vi "write digital out.vi"(8 "error in (no error)":errorcluster) -> ()   [LabVIEW 2015]
uses:
  <vilib>/Rock Robotics/SystemInterfaces/DIO/FPGA_DIOChannel.ctl
  <vilib>/Platform/TimedLoop/XDataNode/timing_clust.ctl
  <vilib>/Platform/TimedLoop/XDataNode/nitl_modes.ctl
  <vilib>/Platform/TimedLoop/XDataNode/wakeup.ctl
  <vilib>/Rock Robotics/WPI/Counter/WPI_CounterDigitalInputToDigitalSource.vi
  <vilib>/Rock Robotics/WPI/Counter/WPI_CounterOpen UpDown Mode.vi
  <vilib>/platform/TimedLoop/XDataNode/XDataNode.xnode
  <vilib>/Platform/TimedLoop/XDataNode/XDNodeRunTimeDep.lvlib
panel:
  out "Value 2":i32
  out "Value":bool
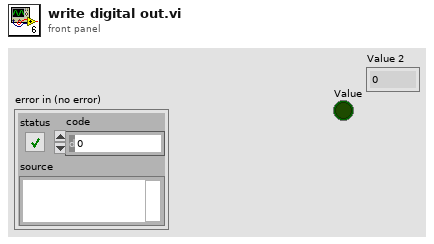
[diagram p1: front panel]
types:
  T1 = typedef "FPGA_DIOChannel.ctl" = enum8{"DIO 0", "DIO 1", "DIO 2", "DIO 3", "DIO 4", "DIO 5", "DIO 6", "DIO 7", "DIO 8", "DIO 9", "DIO MXP 0", "DIO MXP 1", "DIO MXP 2", "DIO MXP 3", "DIO MXP 4", "DIO MXP 5", "DIO MXP 6", "DIO MXP 7", "DIO MXP 8", "DIO MXP 9", "DIO MXP 10", "DIO MXP 11", "DIO MXP 12", "DIO MXP 13", "DIO MXP 14", "DIO MXP 15", "Invalid"}
  T2 = typedef "XDNodeRunTimeDep.lvlib/timing_clust.ctl" = cluster{"Expected End [f-1]":u64, "Actual End [f-1]":u64, "Finished Late? [f-1]":bool, "Expected End [i-1]":u64, "Actual End [i-1]":u64, "Finished Late? [i-1]":bool, "Expected Start [i]":u64, "Actual Start [i]":u64, "Expected Start [f]":u64, "Actual Start [f]":u64, "Source Name":string, "Structure Name":string, "Period":i64, "Deadline":i64, "Offset":i64, "Start":i64, "Priority":i32, "Timeout":i32, "Mode":T3, "Wakeup Reason":T4, "Error":errorcluster, "Source Type":string, "Secondary Source Type":string, "Global End Time":u64, "Global Start Time":u64, "Frame Duration":u64, "Iteration Duration":u64, "Assigned CPU":i32, "I/O Scan Engine Mode":u32}
  T3 = typedef "XDNodeRunTimeDep.lvlib/nitl_modes.ctl" = enum32{"No Change", "Process missed periods, maintain original phase", "Discard missed periods, maintain original phase", "Process missed periods, ignore original phase", "Discard missed periods, ignore original phase"}
  T4 = typedef "XDNodeRunTimeDep.lvlib/wakeup.ctl" = enum32{"Normal", "Aborted", "Asynchronous wakeup", "Timing source error", "Timed loop error", "Timeout"}
  T5 = typedef "WPI_DigitalOutputDevRef.ctl" = cluster{"DIO Channel":T1, "DevStatus":errorcluster}
  T6 = typedef "WPI_DigitalInputDevRef.ctl" = cluster{"DevStatus":errorcluster, "DIO Channel":T1}
  T7 = typedef "FPGA_CounterEncoderSourceConvertionLVSourceType.ctl" = cluster{"DevStatus":errorcluster, "AnalogTriggerMode?":bool, "DigitalMode":cluster{"DIO Channel":T8}, "AnalogTriggerMode":cluster{"AnalogTriggerIndex":T9, "OutputType":T10}}
  T8 = typedef "FPGA_DIODigitalSourceChannel.ctl" = enum8{"DIO 0", "DIO 1", "DIO 2", "DIO 3", "DIO 4", "DIO 5", "DIO 6", "DIO 7", "DIO 8", "DIO 9", "DIO MXP 0", "DIO MXP 1", "DIO MXP 2", "DIO MXP 3", "DIO MXP 4", "DIO MXP 5", "DIO MXP 6", "DIO MXP 7", "DIO MXP 8", "DIO MXP 9", "DIO MXP 10", "DIO MXP 11", "DIO MXP 12", "DIO MXP 13", "DIO MXP 14", "DIO MXP 15", "Disabled"}
  T9 = typedef "FPGA_AnalogTriggerIndex.ctl" = enum8{"Trig 0", "Trig 1", "Trig 2", "Trig 3", "Trig 4", "Trig 5", "Trig 6", "Trig 7", "Invalid"}
  T10 = typedef "FPGA_AnalogTriggerOutType.ctl" = enum16{"InWindow", "TriggerState", "Rising", "Falling"}
  T11 = typedef "WPI_CounterDevRef.ctl" = cluster{"DevStatus":errorcluster, "CntIndex":T12}
  T12 = typedef "FPGA_CounterCtrSystemIndex.ctl" = enum8{"Ctr 0", "Ctr 1", "Ctr 2", "Ctr 3", "Ctr 4", "Ctr 5", "Ctr 6", "Ctr 7", "Invalid"}
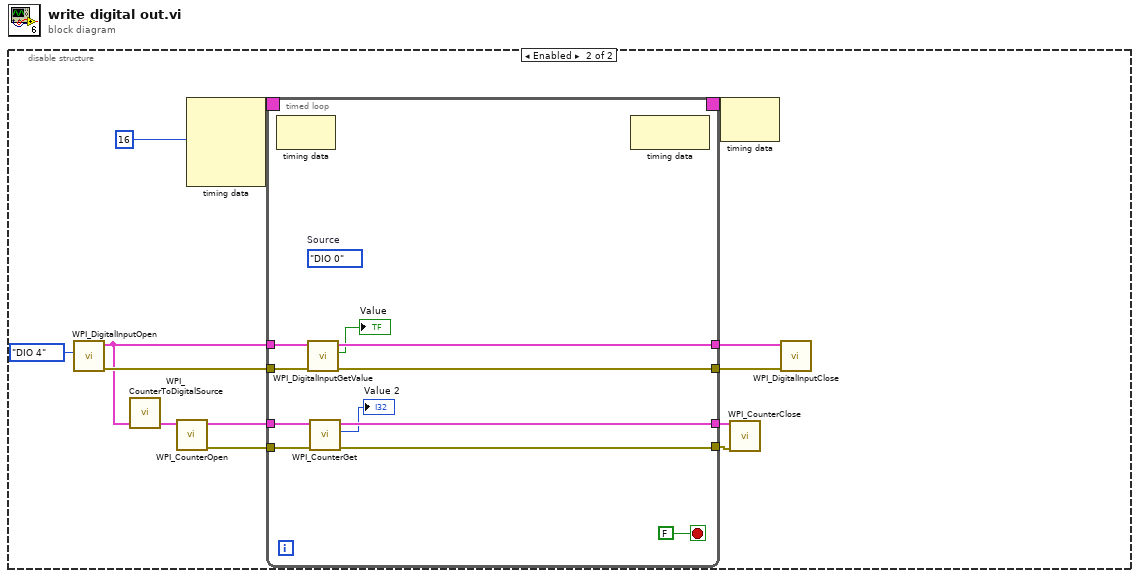
[diagram p0: block diagram]
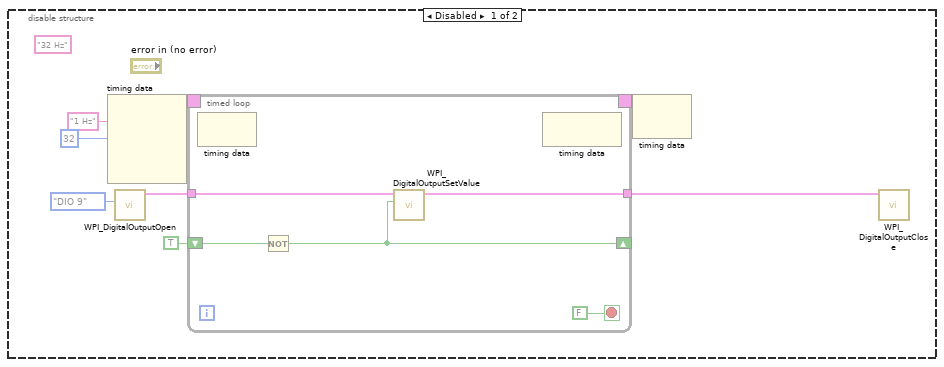
[diagram p2: hidden frame]
diagram:
  n1 = disable-structure shown="Enabled" {
    frame Disabled {
      (unwired) "32 Hz" ("Source Name")
      n2 = node-c288("1 Hz" ("Source Name"), i64 32 ("Period")) -> (w8:T2)  [unwired: 2 in]
      n3 = call <vilib>:"WPI_DigitalOutputOpen.vi"("DIO Channel"=FPGA_DIOChannel."DIO 9") -> ("DigitalOutputDevRef"=w6:T5)  [unwired: 9 in, 1 out]
      n4 = timed-loop {
        timing: w8 -> [_]
        timing-out: [_] -> w7
        tunnel: w6 -> [w12]
        tunnel: [w11] -> w5
        shift-right: [w9] -> _
        shift-left: TRUE -> [w10]
        stop <- FALSE stop-if-true
        n5 = node-c288() -> ()  [unwired: 1 in, 1 out]
        n6 = Not(x=w10) -> (.not. x?=w9:bool)
        n7 = call <vilib>:"WPI_DigitalOutputSetValue.vi"("Value"=w9, "DigitalOutputDevRef"=w12) -> ("DigitalOutputDevRef"=w11:T5)  [unwired: 8 in, 1 out]
        n8 = node-c288() -> ()  [unwired: 1 in, 1 out]
      }
      n9 = node-c288(w7) -> ()  [unwired: 1 out]
      n10 = call <vilib>:"WPI_DigitalOutputClose.vi"("DigitalOutputDevRef"=w5) -> ()  [unwired: 10 in, 1 out]
    }
    frame Enabled {
      n11 = call <vilib>:"WPI_DigitalInputOpen.vi"("DIO Channel"=FPGA_DIOChannel."DIO 4") -> ("error out"=w30:errorcluster, "DigitalInputDevRef"=w25:T6)  [unwired: 9 in]
      n12 = call-poly <vilib>:"WPI_CounterToDigitalSource.vi"("DigitalInputDevRef"=w25) -> ("Digital Source"=w26:T7)  [unwired: 6 out]
      n13 = call-poly <vilib>:"WPI_CounterOpen.vi"("Up Source"=w26) -> ("error out"=w21:errorcluster, "CounterDevRef"=w24:T11)  [unwired: 6 in, 3 out]
      n14 = node-c288(i64 16 ("Period")) -> (w33:T2)  [unwired: 3 in]
      n15 = timed-loop {
        timing: w33 -> [_]
        timing-out: [_] -> w32
        tunnel: w25 -> [w43]
        tunnel: w30 -> [w42]
        tunnel: [w41] -> w28
        tunnel: [w39] -> w29
        tunnel: w24 -> [w38]
        tunnel: [w37] -> w23
        tunnel: [w36] -> w22
        tunnel: w21 -> [w34]
        stop <- FALSE stop-if-true
        (unwired) FPGA_DIOChannel."DIO 0"  # Source
        n16 = node-c288() -> ()  [unwired: 1 in, 1 out]
        n17 = call <vilib>:"WPI_DigitalInputGetValue.vi"("error in (no error)"=w42, "DigitalInputDevRef"=w43) -> ("error out"=w39:errorcluster, "Value"=→"Value":bool, "DigitalInputDevRef"=w41:T6)  [unwired: 7 in]
        n18 = call <vilib>:"WPI_CounterGet.vi"("error in (no error)"=w34, "CounterDevRef in"=w38) -> ("error out"=w36:errorcluster, "Value"=→"Value 2":i32, "CounterDevRef out"=w37:T11)  [unwired: 4 in, 3 out]
        n19 = node-c288() -> ()  [unwired: 1 in, 1 out]
      }
      n20 = node-c288(w32) -> ()  [unwired: 1 out]
      n21 = call <vilib>:"WPI_CounterClose.vi"("error in (no error)"=w22, "CounterDevRef"=w23) -> ()  [unwired: 9 in, 1 out]
      n22 = call <vilib>:"WPI_DigitalInputClose.vi"("error in (no error)"=w29, "DigitalInputDevRef"=w28) -> ()  [unwired: 9 in, 1 out]
    }
  }
